vi "Prefilter.60Hz_Notch.vi"(8 "error in (no error)":errorcluster, 11 "Instrument.DAQ":refnum<class "Instrument.DAQ.lvclass">) -> (0 "error out":errorcluster, 3 "Instrument.DAQ out":refnum<class "Instrument.DAQ.lvclass">)   [LabVIEW 2019, in "Instrument.Lockin.lvlib" / "Instrument.DAQ.lvclass"]
uses:
  Instrument.DAQ.lvclass
  Instrument.DAQ.lvclass/Instrument.DAQ.ctl
  <vilib>/addons/Digital Filter Design/NI_DigFilterLicensed.lvlib
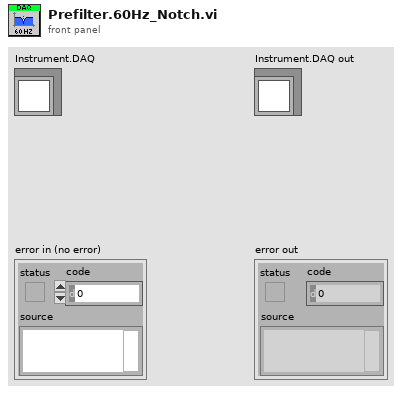
[diagram p1: front panel]
types:
  T1 = typedef "NI_DigFilterLicensed.lvlib/DFD Filter Obj.ctl" = cluster{"mSRate_Fs":dbl, "mSRate_Version":string, "mSRate_Comments":string, "mSRate_OrgCoef":T2, "mSRate_CurCoef":T2, "mSRate_Quantized?":bool, "mSRate_QCoef":T2, "mSRate_QSettings":T4[], "mSRate_Order":i32, "mSRate_Scaling":cluster{"mSRate_ScaleByPowerOf2?":bool, "mSRate_ScaleType":T6}}
  T2 = typedef "NI_DigFilterLicensed.lvlib/DFD Filter Coef.ctl" = cluster{"type":T3, "gain":dbl, "coef a (k)":dbl[], "coef b (v)":dbl[]}
  T3 = typedef "NI_DigFilterLicensed.lvlib/DFD Filter Structure Type Selector.ctl" = enum16{"Undefined", "FIR Direct Form", "FIR Direct Form Transposed", "FIR Symmetric", "FIR Antisymmetric", "IIR Direct Form I", "IIR Direct Form I Transposed", "IIR Direct Form II", "IIR Direct Form II Transposed", "IIR Cascaded Second Order Sections Form I", "IIR Cascaded Second Order Sections Form I Transposed", "IIR Cascaded Second Order Sections Form II", "IIR Cascaded Second Order Sections Form II Transposed", "Lattice Allpass (basic sections)", "Lattice Allpass (one multiplier sections)", "Lattice Allpass (normalized sections)", "Lattice AR (basic sections)", "Lattice AR (one multiplier sections)", "Lattice AR (normalized sections)", "Lattice MA (minimum phase)", "Lattice MA (maximum phase)", "Lattice ARMA (basic sections)", "Lattice ARMA (one multiplier sections)", "Lattice ARMA (normalized sections)"}
  T4 = typedef "NI_DigFilterLicensed.lvlib/dfd_Internal Quantization Settings.ctl" = cluster{"source":T5, "wl":i16, "iwl":i16, "overflow mode":enum16{"Saturation", "Wrap"}, "rounding mode":enum16{"Nearest", "Truncation"}, "signed?":bool}
  T5 = typedef "NI_DigFilterLicensed.lvlib/dfd_Internal Quantization Srcs.ctl" = u16
  T6 = typedef "NI_DigFilterLicensed.lvlib/DFD Coef Norm Type.ctl" = enum16{"No Norm", "Time Domain 1-Norm", "Time Domain 2-Norm", "Time Domain Inf-Norm"}
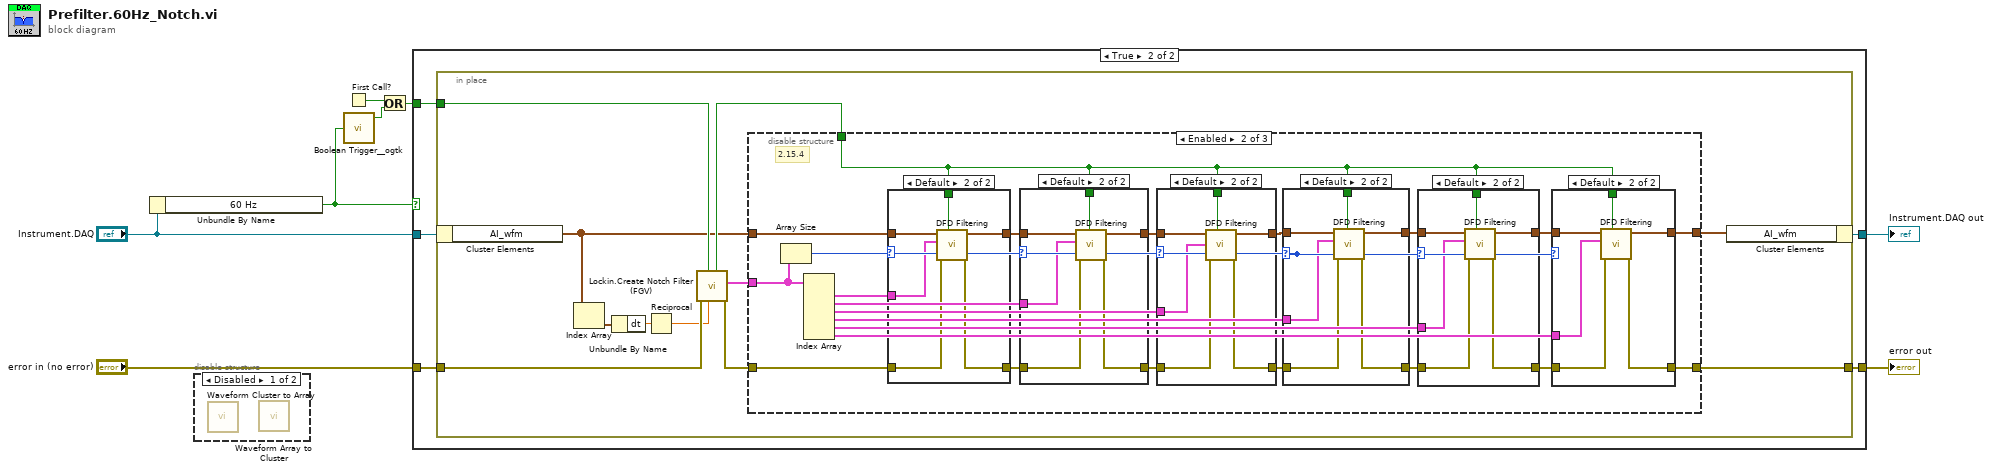
[diagram p0: block diagram]
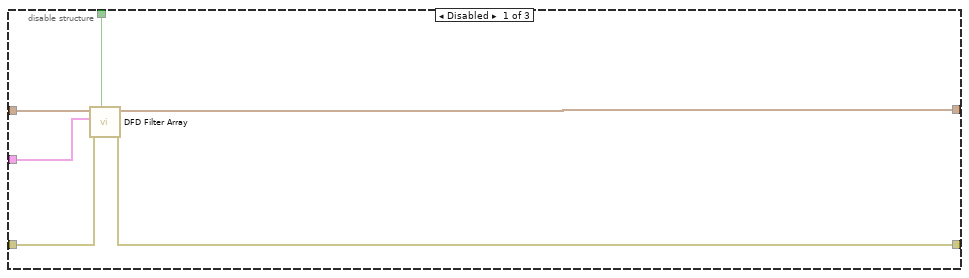
[diagram p3: hidden frame]
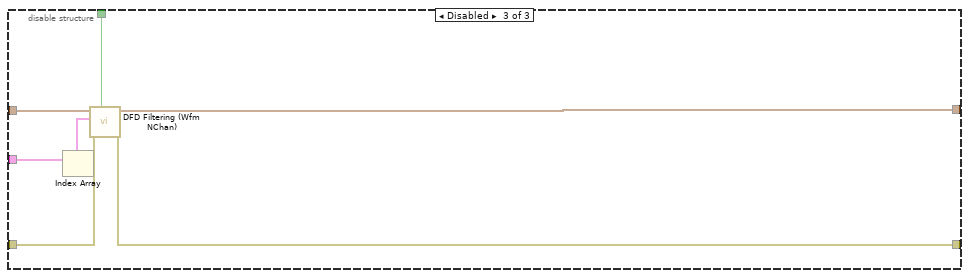
[diagram p10: hidden frame]
diagram:
  n1 = Unbundle By Name("Instrument.DAQ") -> ("60 Hz"=w2:bool)
  n2 = disable-structure shown="Disabled" {
    frame Disabled {
      n3 = call "Waveform Cluster to Array.vi"() -> ()  [unwired: 10 in, 2 out]
      n4 = call "Waveform Array to Cluster.vi"() -> ()  [unwired: 11 in, 1 out]
    }
    frame Enabled {
    }
  }
  n5 = First Call?() -> (First Call?: T/F=w4:bool)
  n6 = call <userlib>:"Boolean Trigger__ogtk.vi"("Boolean Input"=w2) -> ("Rising Edge"=w1:bool)  [unwired: 1 in, 1 out]
  n7 = Or(x=w4, y=w1) -> (x .or. y?=w3:bool)
  n8 = case shown="True" w2 {
    tunnel: "error in (no error)" -> [w9 w15]
    tunnel: [w9 w14] -> w7
    tunnel: "Instrument.DAQ" -> [w10 w12]
    tunnel: [w10 w11] -> w6
    tunnel: w3 -> [_ w13]
    frame False {
    }
    frame True {
      n9 = in-place {
        in-place-border: w15 -> [w26]
        in-place-border: [w23] -> w14
        in-place-border: w13 -> [w20]
        n10 = in-place-cluster #1(w12) -> ("AI_wfm"=w17:waveform(dbl)[])
        n11 = Index Array(array=w17) -> (element=w24:waveform(dbl))  [unwired: 1 in]
        n12 = Unbundle By Name(w24) -> ("dt"=w25:dbl)
        n13 = Reciprocal(x=w25) -> (1/x=w21:dbl)
        n14 = call "Lockin.Create Notch Filter (FGV).vi"("fs (Hz)"=w21, "init [F]"=w20, "error in (no error)"=w26) -> ("error out"=w18:errorcluster, "filters out"=w22:T1[], "init?"=w19:bool)  [unwired: 6 in]
        n15 = disable-structure shown="Enabled" {
          disable-tunnel: [w32 w43 w109] -> w16
          disable-tunnel: [w31 w45 w106] -> w23
          disable-tunnel: w18 -> [w30 w40 w107]
          disable-tunnel: w17 -> [w29 w44 w110]
          disable-tunnel: w22 -> [w28 w39 w105]
          disable-tunnel: w19 -> [w27 w42 w108]
          frame Disabled {
            n16 = call "DFD Filter Array.vi"("init (F)"=w27, "error in (no error)"=w30, "filters"=w28, "signal in"=w29) -> ("error out"=w31:errorcluster, "signal out"=w32:waveform(dbl)[])  [unwired: 6 in]
          }
          frame Enabled {
            # "2.15.4"
            n17 = Array Size(array=w39) -> (size(s)=w41:i32)
            n18 = Index Array(array=w39) -> (element #1=w38:T1, element #2=w37:T1, element #3=w36:T1, element #4=w35:T1, element #5=w34:T1, element #6=w33:T1)  [unwired: 6 in]
            n19 = case shown="Default" w41 {
              tunnel: [w57 w63] -> w52
              tunnel: [w56 w62] -> w53
              tunnel: w44 -> [w57 w61]
              tunnel: w42 -> [_ w60]
              tunnel: w40 -> [w56 w59]
              tunnel: w38 -> [_ w58]
              frame 0 {
              }
              frame Default {
                n20 = call-poly <vilib>:"DFD Filtering.vi"("init? (F)"=w60, "error in (no error)"=w59, "filter"=w58, "signal in"=w61) -> ("error out"=w62:errorcluster, "signal out"=w63:waveform(dbl)[])  [unwired: 6 in]
              }
            }
            n21 = case shown="Default" w41 {
              tunnel: [w65 w71] -> w46
              tunnel: [w64 w70] -> w51
              tunnel: w52 -> [w65 w69]
              tunnel: w53 -> [w64 w68]
              tunnel: w42 -> [_ w67]
              tunnel: w37 -> [_ w66]
              frame 0, 1 {
              }
              frame Default {
                n22 = call-poly <vilib>:"DFD Filtering.vi"("init? (F)"=w67, "error in (no error)"=w68, "filter"=w66, "signal in"=w69) -> ("error out"=w70:errorcluster, "signal out"=w71:waveform(dbl)[])  [unwired: 6 in]
              }
            }
            n23 = case shown="Default" w41 {
              tunnel: w46 -> [w72 w79]
              tunnel: [w72 w78] -> w47
              tunnel: [w73 w77] -> w49
              tunnel: w51 -> [w73 w76]
              tunnel: w42 -> [_ w75]
              tunnel: w36 -> [_ w74]
              frame 0..2 {
              }
              frame Default {
                n24 = call-poly <vilib>:"DFD Filtering.vi"("init? (F)"=w75, "error in (no error)"=w76, "filter"=w74, "signal in"=w79) -> ("error out"=w77:errorcluster, "signal out"=w78:waveform(dbl)[])  [unwired: 6 in]
              }
            }
            n25 = case shown="Default" w41 {
              tunnel: w47 -> [w81 w87]
              tunnel: [w81 w86] -> w48
              tunnel: w49 -> [w80 w84]
              tunnel: [w80 w85] -> w50
              tunnel: w42 -> [_ w83]
              tunnel: w35 -> [_ w82]
              frame 0..3 {
              }
              frame Default {
                n26 = call-poly <vilib>:"DFD Filtering.vi"("init? (F)"=w83, "error in (no error)"=w84, "filter"=w82, "signal in"=w87) -> ("error out"=w85:errorcluster, "signal out"=w86:waveform(dbl)[])  [unwired: 6 in]
              }
            }
            n27 = case shown="Default" w41 {
              tunnel: [w88 w95] -> w55
              tunnel: w48 -> [w89 w94]
              tunnel: w50 -> [w88 w92]
              tunnel: [w89 w93] -> w54
              tunnel: w42 -> [_ w91]
              tunnel: w34 -> [_ w90]
              frame 0..4 {
              }
              frame Default {
                n28 = call-poly <vilib>:"DFD Filtering.vi"("init? (F)"=w91, "error in (no error)"=w92, "filter"=w90, "signal in"=w94) -> ("error out"=w95:errorcluster, "signal out"=w93:waveform(dbl)[])  [unwired: 6 in]
              }
            }
            n29 = case shown="Default" w41 {
              tunnel: [w96 w103] -> w45
              tunnel: w54 -> [w97 w102]
              tunnel: w55 -> [w96 w100]
              tunnel: [w97 w101] -> w43
              tunnel: w42 -> [_ w99]
              tunnel: w33 -> [_ w98]
              frame 0..5 {
              }
              frame Default {
                n30 = call-poly <vilib>:"DFD Filtering.vi"("init? (F)"=w99, "error in (no error)"=w100, "filter"=w98, "signal in"=w102) -> ("error out"=w103:errorcluster, "signal out"=w101:waveform(dbl)[])  [unwired: 6 in]
              }
            }
          }
          frame Disabled {
            n31 = Index Array(array=w105) -> (element=w104:T1)  [unwired: 1 in]
            n32 = call <vilib>:"DFD Filtering (Wfm NChan).vi"("init? (F)"=w108, "error in (no error)"=w107, "filter"=w104, "signal in"=w110) -> ("error out"=w106:errorcluster, "signal out"=w109:waveform(dbl)[])  [unwired: 6 in]
          }
        }
        n33 = in-place-cluster #1("AI_wfm"=w16) -> (w11:refnum<class "Instrument.DAQ.lvclass">)
      }
    }
  }
  "error out" <- w7
  "Instrument.DAQ out" <- w6
